vi "ReceiveTriggerCommand.vi"(8 "error in (no error)":errorcluster, 9 "Args":string[](array[string]), 10 "Command":string, 11 "TektronixDPOSimple in":refnum<class "Tektronix MDO MSO DPO.lvclass">) -> (0 "error out":errorcluster, 2 "new commands":string, 3 "TektronixDPOSimple out":refnum<class "Tektronix MDO MSO DPO.lvclass">)   [LabVIEW 2020, in "Tektronix MDO MSO DPO.lvclass"]
uses:
  Tektronix MDO MSO DPO.lvclass
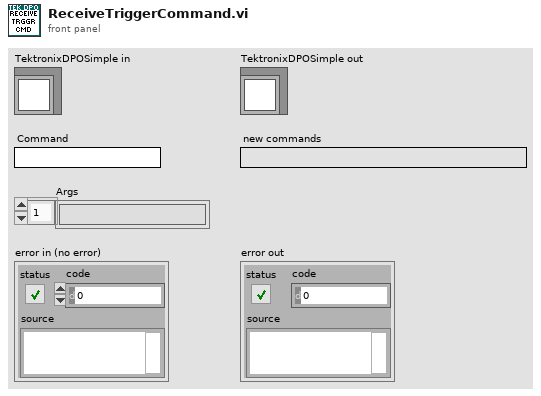
[diagram p1: front panel]
types:
  T1 = typedef "TriggerCluster.ctl" = cluster{"Mode":T2, "Source":u16, "Coupling":u16, "Level":dbl, "Slope":u16}
  T2 = typedef "TriggerModes.ctl" = u16
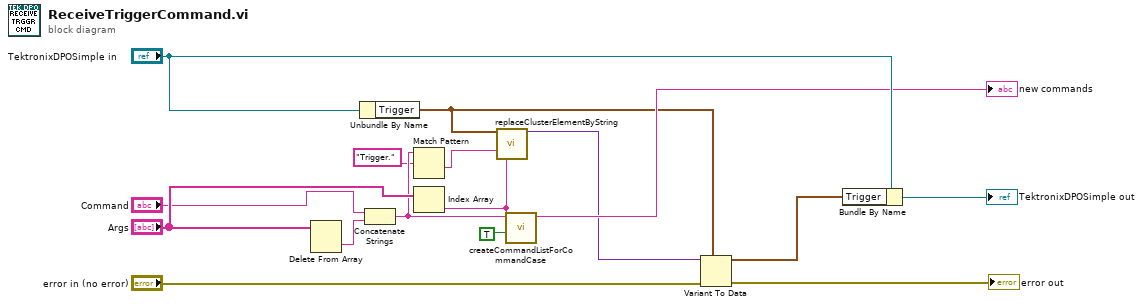
[diagram p0: block diagram]
diagram:
  n1 = Delete From Array(array="Args") -> (deleted portion=w8:string)  [unwired: 2 in, 1 out]
  n2 = Unbundle By Name("TektronixDPOSimple in") -> ("Trigger"=w6:T1)
  n3 = Concatenate Strings("Command", w8) -> (w4:string)
  n4 = Match Pattern(string=w4, regular expression="Trigger." ("search string")) -> (after substring=w1:string)  [unwired: 1 in, 3 out]
  n5 = Index Array(array="Args") -> (element=w5:string)  [unwired: 1 in]
  n6 = call "replaceClusterElementByString.vi"("cluster in"=w6, "Command"=w1, "setvalue"=w5) -> ("cluster out"=w7:variant)  [unwired: 10 in, 2 out]
  n7 = call "createCommandListForCommandCase.vi"("immediate Check (only once)"=TRUE, "setvalue"=w5, "command"=w4) -> ("new commands"=→"new commands":string)  [unwired: 8 in]
  n8 = Variant To Data(error in="error in (no error)", type=w6, Variant=w7) -> (data=w14:T1, error out=→"error out":errorcluster)
  n9 = Bundle By Name(cluster="TektronixDPOSimple in", "Trigger"=w14) -> (→"TektronixDPOSimple out":refnum<class "Tektronix MDO MSO DPO.lvclass">)
